vi "4155C Transfer-FPP Config SMUs v2.0.vi"(0 "VISA resource name in":refnum<visa-resource-name>, 1 "Pulse period":dbl=0.005 min=0.005 max=1.0 step=0.0001 format="%.4f", 2 "FPP - Drain":u32(ring)=1 items=["SMU1  ", "SMU2  ", "SMU3  ", "SMU4  ", "SMU5  ", "SMU6  "], 3 "Pulse width":dbl=0.0005 min=0.0005 max=0.1 step=0.0001 format="%.4f", 4 "Base voltage":dbl format="%^.4e", 5 "error in (no error)":errorcluster, 6 "sweep method":u16(ring) items=["Continuous", "Pulsed"], 7 "FPP - Probe 1":u32(ring) items=["SMU1  ", "SMU2  ", "SMU3  ", "SMU4  ", "SMU5  ", "SMU6  "], 8 "FPP - Gate":u32(ring)=2 items=["SMU1  ", "SMU2  ", "SMU3  ", "SMU4  ", "SMU5  ", "SMU6  "], 9 "FPP - Probe 2":u32(ring)=3 items=["SMU1  ", "SMU2  ", "SMU3  ", "SMU4  ", "SMU5  ", "SMU6  "], 10 "Gate mode":u16(ring) items=["Auto", "Limited", "Fixed"], 11 "Source/drain mode":u16(ring) items=["Auto", "Limited", "Fixed"], 12 "Gate Range":u8(slide)=6 max=11 scale=0.0..11.0, 13 "Source/drain Range":u8(slide)=6 max=11 scale=0.0..11.0, 15 "FPP - Source":u32(ring) items=["VSU1  ", "VSU2  "]) -> (14 "VISA Resource Name out":refnum<visa-resource-name>, 19 "error out":errorcluster)   [LabVIEW 2016]
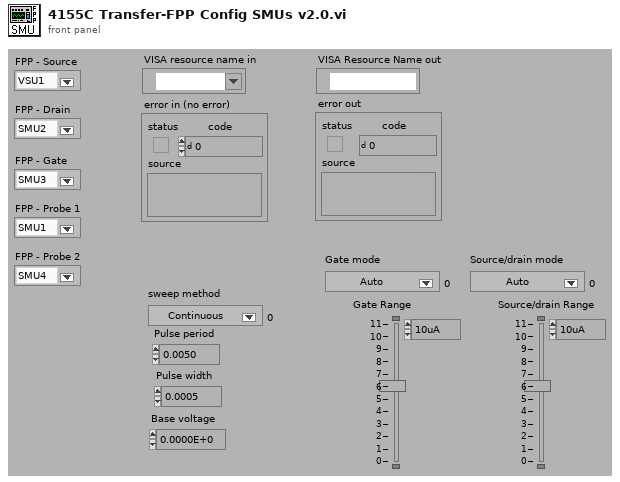
[diagram p1: front panel]
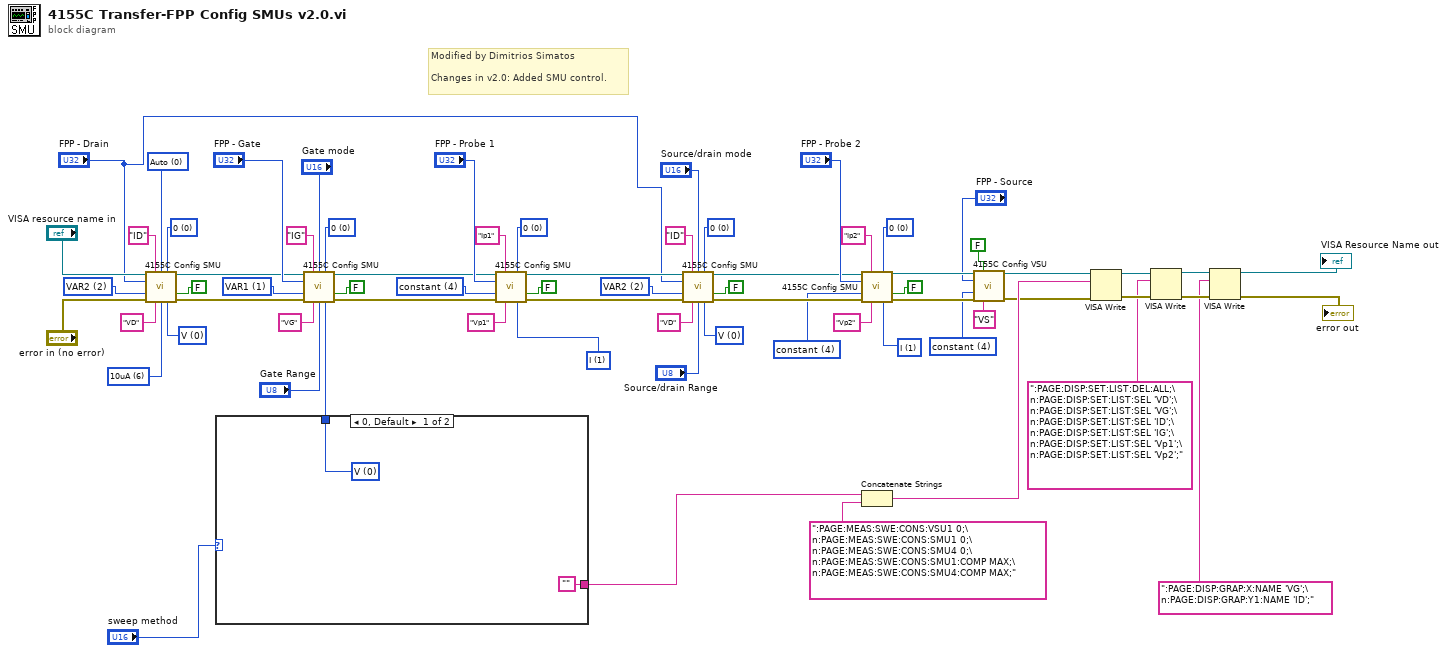
[diagram p0: block diagram]
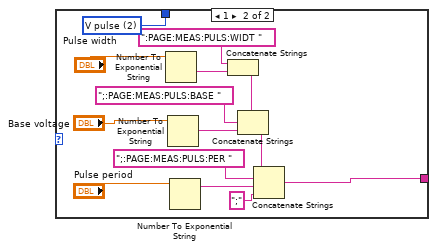
[diagram p2: hidden frame]
diagram:
  w15 = u32 4 items=["disabled  ", "VAR1  ", "VAR2  ", "VAR1'  ", "constant  "] ("function")
  w22 = u32 4 items=["disabled  ", "VAR1  ", "VAR2  ", "VAR1'  ", "constant  "] ("function")
  w26 = u32 1 items=["V  ", "I  ", "V pulse  ", "I pulse  ", "  common  "] ("mode")
  w27 = u16 0 items=["Auto", "Limited", "Fixed"] ("Range mode")
  w28 = u8 6 items=["10fA  ", "100fA  ", "1nA  ", "10nA", "100nA", "1uA", "10uA", "100uA", "1mA", "10mA", "100mA", "1A"] ("Range")
  w33 = u32 2 items=["disabled  ", "VAR1  ", "VAR2  ", "VAR1'  ", "constant  "] ("function")
  w35 = u32 0 items=["0  ", "10K Ohms  ", "100K Ohms  ", "1M Ohms  "] ("series resistance *")
  w36 = u32 0 items=["V  ", "I  ", "V pulse  ", "I pulse  ", "  common  "] ("mode")
  w50 = u32 0 items=["0  ", "10K Ohms  ", "100K Ohms  ", "1M Ohms  "] ("series resistance *")
  w55 = u32 0 items=["V  ", "I  ", "V pulse  ", "I pulse  ", "  common  "] ("mode")
  w56 = u32 0 items=["0  ", "10K Ohms  ", "100K Ohms  ", "1M Ohms  "] ("series resistance *")
  w58 = u32 2 items=["disabled  ", "VAR1  ", "VAR2  ", "VAR1'  ", "constant  "] ("function")
  w61 = u32 0 items=["0  ", "10K Ohms  ", "100K Ohms  ", "1M Ohms  "] ("series resistance *")
  w63 = u32 4 items=["disabled  ", "VAR1  ", "VAR2  ", "VAR1'  ", "constant  "] ("function")
  w40 = u32 1 items=["V  ", "I  ", "V pulse  ", "I pulse  ", "  common  "] ("mode")
  w67 = u32 0 items=["0  ", "10K Ohms  ", "100K Ohms  ", "1M Ohms  "] ("series resistance *")
  w69 = u32 1 items=["disabled  ", "VAR1  ", "VAR2  ", "VAR1'  ", "constant  "] ("function")
  # "Modified by Dimitrios Simatos\n\nChanges in v2.0: Added SMU control."
  n1 = call "4155C Config SMU.vi"("VISA session"="VISA resource name in", "I name (max 6 chars)"="ID", "Range mode"=w27, "series resistance *"=w35, "unit to configure"="FPP - Drain", "function"=w33, "standby"=FALSE, "error in (no error)"="error in (no error)", "V name (max 6 chars)"="VD", "Range"=w28, "mode"=w36) -> ("dup VISA resource name"=w30:refnum<visa-resource-name>, "error out"=w31:errorcluster)  [unwired: 3 in]
  n2 = case shown="0, Default" "sweep method" {
    tunnel: [w72 w86] -> w39
    tunnel: ["" w77] -> w25
    frame 0, Default {
      w72 = u32 0 items=["V  ", "I  ", "V pulse  ", "I pulse  ", "  common  "] ("mode")
    }
    frame 1 {
      w86 = u32 2 items=["V  ", "I  ", "V pulse  ", "I pulse  ", "  common  "] ("mode")
      n3 = Number To Exponential String(number="Pulse width") -> (E-format string=w85:string)  [unwired: 3 in]
      n4 = Number To Exponential String(number="Base voltage") -> (E-format string=w81:string)  [unwired: 3 in]
      n5 = Number To Exponential String(number="Pulse period") -> (E-format string=w78:string)  [unwired: 3 in]
      n6 = Concatenate Strings(":PAGE:MEAS:PULS:WIDT " ("Substring"), w85) -> (w83:string)
      n7 = Concatenate Strings(w83, ";:PAGE:MEAS:PULS:BASE " ("Substring"), w81) -> (w79:string)
      n8 = Concatenate Strings(w79, ";:PAGE:MEAS:PULS:PER " ("Substring"), w78, ";" ("Substring")) -> (w77:string)
    }
  }
  n9 = call "4155C Config SMU.vi"("VISA session"=w30, "I name (max 6 chars)"="IG", "Range mode"="Gate mode", "series resistance *"=w67, "unit to configure"="FPP - Gate", "function"=w69, "standby"=FALSE, "error in (no error)"=w31, "V name (max 6 chars)"="VG", "Range"="Gate Range", "mode"=w39) -> ("dup VISA resource name"=w47:refnum<visa-resource-name>, "error out"=w46:errorcluster)  [unwired: 3 in]
  n10 = call "4155C Config SMU.vi"("VISA session"=w47, "I name (max 6 chars)"="Ip1", "series resistance *"=w61, "unit to configure"="FPP - Probe 1", "function"=w63, "standby"=FALSE, "error in (no error)"=w46, "V name (max 6 chars)"="Vp1", "mode"=w40) -> ("dup VISA resource name"=w44:refnum<visa-resource-name>, "error out"=w45:errorcluster)  [unwired: 5 in]
  n11 = call "4155C Config SMU.vi"("VISA session"=w44, "I name (max 6 chars)"="ID", "Range mode"="Source/drain mode", "series resistance *"=w56, "unit to configure"="FPP - Drain", "function"=w58, "standby"=FALSE, "error in (no error)"=w45, "V name (max 6 chars)"="VD", "Range"="Source/drain Range", "mode"=w55) -> ("dup VISA resource name"=w43:refnum<visa-resource-name>, "error out"=w42:errorcluster)  [unwired: 3 in]
  n12 = call "4155C Config SMU.vi"("VISA session"=w43, "I name (max 6 chars)"="Ip2", "series resistance *"=w50, "unit to configure"="FPP - Probe 2", "function"=w22, "standby"=FALSE, "error in (no error)"=w42, "V name (max 6 chars)"="Vp2", "mode"=w26) -> ("dup VISA resource name"=w20:refnum<visa-resource-name>, "error out"=w21:errorcluster)  [unwired: 5 in]
  n13 = Concatenate Strings(w25, ":PAGE:MEAS:SWE:CONS:VSU1 0;\n:PAGE:MEAS:SWE:CONS:SMU1 0;\n:PAGE:MEAS:SWE:CONS:SMU4 0;\n:PAGE:MEAS:SWE:CONS:SMU1:COMP MAX;\n:PAGE:MEAS:SWE:CONS:SMU4:COMP MAX;" ("write buffer (\"\")")) -> (w23:string)
  n14 = call "4155C Config VSU.vi"("VISA session"=w20, "standby"=FALSE, "unit to configure"="FPP - Source", "function"=w15, "error in (no error)"=w21, "V name (max 6 chars)"="VS") -> ("dup VISA resource name"=w18:refnum<visa-resource-name>, "error out"=w19:errorcluster)  [unwired: 8 in]
  n15 = VISA Write(VISA resource name=w18, write buffer=w23, error in (no error)=w19) -> (VISA resource name out=w9:refnum<visa-resource-name>, error out=w4:errorcluster)  [unwired: 1 out]
  n16 = VISA Write(VISA resource name=w9, write buffer=":PAGE:DISP:SET:LIST:DEL:ALL;\n:PAGE:DISP:SET:LIST:SEL 'VD';\n:PAGE:DISP:SET:LIST:SEL 'VG';\n:PAGE:DISP:SET:LIST:SEL 'ID';\n:PAGE:DISP:SET:LIST:SEL 'IG';\n:PAGE:DISP:SET:LIST:SEL 'Vp1';\n:PAGE:DISP:SET:LIST:SEL 'Vp2';" ("write buffer (\"\")"), error in (no error)=w4) -> (VISA resource name out=w8:refnum<visa-resource-name>, error out=w5:errorcluster)  [unwired: 1 out]
  n17 = VISA Write(VISA resource name=w8, write buffer=":PAGE:DISP:GRAP:X:NAME 'VG';\n:PAGE:DISP:GRAP:Y1:NAME 'ID';" ("write buffer (\"\")"), error in (no error)=w5) -> (VISA resource name out=→"VISA Resource Name out":refnum<visa-resource-name>, error out=→"error out":errorcluster)  [unwired: 1 out]
